vi "Drop Sand.vi"(5 "Y in":i32, 7 "X in":i32, 8 "Bottom in":i32[](array[numeric]), 9 "Top in":i32[](array[numeric]), 10 "Right in":i32[](array[numeric]), 11 "Left in":i32[](array[numeric])) -> (0 "Bottom out":i32[](array[numeric]), 1 "Top out":i32[](array[numeric]), 2 "Right out":i32[](array[numeric]), 3 "Left out":i32[](array[numeric]), 4 "falling forever?":bool)   [LabVIEW 2021, in "d14.lvlib"]
uses:
  d14.lvlib
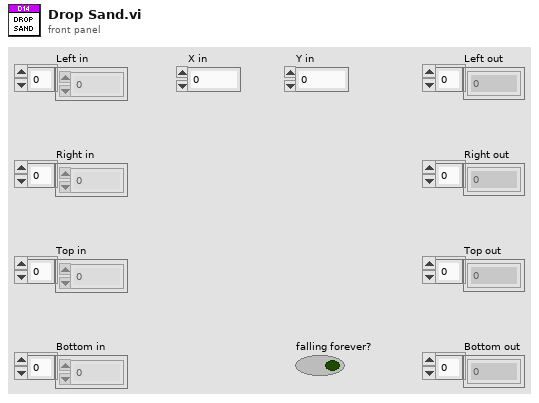
[diagram p1: front panel]
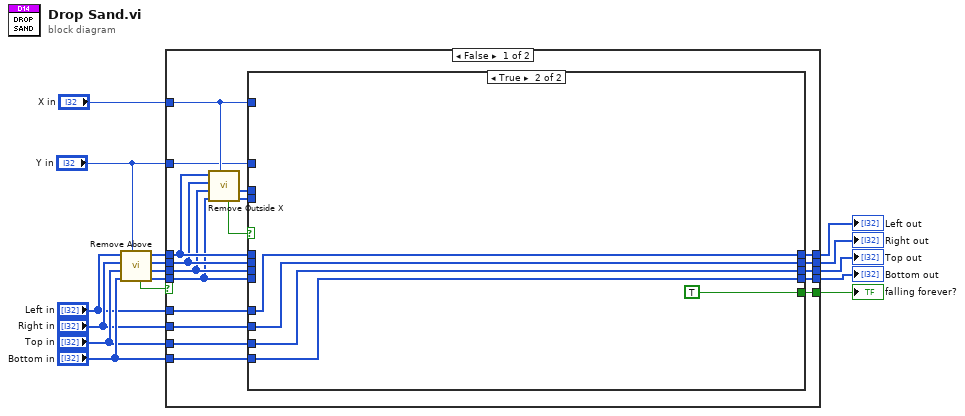
[diagram p0: block diagram]
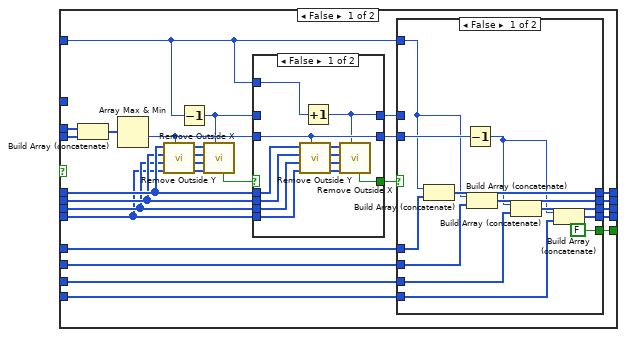
[diagram p2: hidden frame]
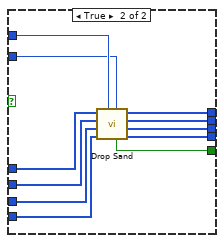
[diagram p3: hidden frame]
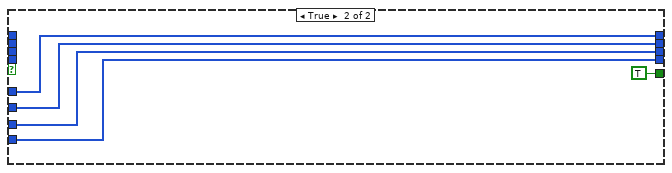
[diagram p5: hidden frame]
diagram:
  n1 = call "Remove Above.vi"("Y in"="Y in", "Bottom in"="Bottom in", "Top in"="Top in", "Right in"="Right in", "Left in"="Left in") -> ("Bottom out"=w12:i32[], "Top out"=w13:i32[], "Right out"=w14:i32[], "Left out"=w15:i32[], "empty?"=w9:bool)  [unwired: 2 in]
  n2 = case shown="False" w9 {
    tunnel: "X in" -> [w34 _]
    tunnel: w15 -> [w33 _]
    tunnel: w14 -> [w32 _]
    tunnel: w13 -> [w31 _]
    tunnel: w12 -> [w30 _]
    tunnel: "Y in" -> [w29 _]
    tunnel: [w28 TRUE ("falling forever?")] -> w10
    tunnel: [w24 w108] -> w8
    tunnel: [w23 w107] -> w7
    tunnel: [w22 w105] -> w5
    tunnel: [w21 w106] -> w6
    tunnel: "Bottom in" -> [w20 w105]
    tunnel: "Top in" -> [w19 w106]
    tunnel: "Right in" -> [w18 w107]
    tunnel: "Left in" -> [w17 w108]
    frame False {
      n3 = call "Remove Outside X.vi"("X in"=w34, "Bottom in"=w30, "Top in"=w31, "Right in"=w32, "Left in"=w33) -> ("Bottom out"=w26:i32[], "Top out"=w27:i32[], "empty?"=w25:bool)  [unwired: 2 in, 2 out]
      n4 = case shown="True" w25 {
        tunnel: w34 -> [w39 _]
        tunnel: w33 -> [w53 _]
        tunnel: w32 -> [w52 _]
        tunnel: w31 -> [w51 _]
        tunnel: w30 -> [w50 _]
        tunnel: w29 -> [_ _]
        tunnel: [w46 TRUE ("falling forever?")] -> w28
        tunnel: w27 -> [w57 _]
        tunnel: w26 -> [w56 _]
        tunnel: [w45 w103] -> w24
        tunnel: [w44 w102] -> w23
        tunnel: [w43 w101] -> w21
        tunnel: [w42 w100] -> w22
        tunnel: w20 -> [w38 w100]
        tunnel: w19 -> [w37 w101]
        tunnel: w18 -> [w36 w102]
        tunnel: w17 -> [w35 w103]
        frame False {
          n5 = Build Array (concatenate)(w57, w56) -> (w55:i32[])
          n6 = Array Max & Min(array=w55) -> (min value=w49:i32)  [unwired: 3 out]
          n7 = call "Remove Outside Y.vi"("Y in"=w49, "Bottom in"=w50, "Top in"=w51, "Right in"=w52, "Left in"=w53) -> ("Bottom out"=w61:i32[], "Top out"=w60:i32[], "Right out"=w59:i32[], "Left out"=w58:i32[])  [unwired: 2 in, 1 out]
          n8 = Decrement(x=w39) -> (x-1=w41:i32)
          n9 = call "Remove Outside X.vi"("X in"=w41, "Bottom in"=w61, "Top in"=w60, "Right in"=w59, "Left in"=w58) -> ("empty?"=w54:bool)  [unwired: 2 in, 4 out]
          n10 = case shown="False" w54 {
            selector: w54 -> [_ w99]
            tunnel: w53 -> [w90 _]
            tunnel: w52 -> [w89 _]
            tunnel: w51 -> [w88 _]
            tunnel: w50 -> [w87 _]
            tunnel: w39 -> [w92 _]
            tunnel: w49 -> [w86 w98]
            tunnel: [w91 w99] -> w48
            tunnel: [w86 w98] -> w47
            tunnel: w41 -> [_ w97]
            tunnel: [w85 w97] -> w40
            frame False {
              n11 = call "Remove Outside Y.vi"("Y in"=w86, "Bottom in"=w87, "Top in"=w88, "Right in"=w89, "Left in"=w90) -> ("Bottom out"=w93:i32[], "Top out"=w96:i32[], "Right out"=w95:i32[], "Left out"=w94:i32[])  [unwired: 2 in, 1 out]
              n12 = Increment(x=w92) -> (x+1=w85:i32)
              n13 = call "Remove Outside X.vi"("X in"=w85, "Bottom in"=w93, "Top in"=w96, "Right in"=w95, "Left in"=w94) -> ("empty?"=w91:bool)  [unwired: 2 in, 4 out]
            }
            frame True {
            }
          }
          n14 = case shown="False" w48 {
            tunnel: w40 -> [_ w84]
            tunnel: w47 -> [w68 w83]
            tunnel: [FALSE ("falling forever?") w82] -> w46
            tunnel: [w73 w81] -> w45
            tunnel: [w72 w80] -> w44
            tunnel: [w71 w79] -> w43
            tunnel: [w70 w78] -> w42
            tunnel: w39 -> [w66 _]
            tunnel: w38 -> [w65 w74]
            tunnel: w37 -> [w64 w75]
            tunnel: w36 -> [w63 w76]
            tunnel: w35 -> [w62 w77]
            frame False {
              n15 = Build Array (concatenate)(w66, w62) -> (w73:i32[])
              n16 = Decrement(x=w68) -> (x-1=w67:i32)
              n17 = Build Array (concatenate)(w66, w63) -> (w72:i32[])
              n18 = Build Array (concatenate)(w67, w64) -> (w71:i32[])
              n19 = Build Array (concatenate)(w67, w65) -> (w70:i32[])
            }
            frame True {
              n20 = call "Drop Sand.vi"("Y in"=w83, "X in"=w84, "Bottom in"=w74, "Top in"=w75, "Right in"=w76, "Left in"=w77) -> ("Bottom out"=w78:i32[], "Top out"=w79:i32[], "Right out"=w80:i32[], "Left out"=w81:i32[], "falling forever?"=w82:bool)  [unwired: 1 in]
            }
          }
        }
        frame True {
        }
      }
    }
    frame True {
    }
  }
  "falling forever?" <- w10
  "Left out" <- w8
  "Right out" <- w7
  "Top out" <- w6
  "Bottom out" <- w5
